vi "Launch Game.vi"() -> ()   [LabVIEW 2020]
uses:
  Main Reversi.vi
  Reversi.lvclass
panel:
  in  "Wait per Turn (ms)":u32=200 max=1000
  in  "Close":bool
  in  "Start":bool
  in  "Game Mode":T1(ring)=enum."Challenge Matches (All Players)"
  in  "Games Per Match":u32=1 min=1 max=1000
  # "Wait is changeable during the game."
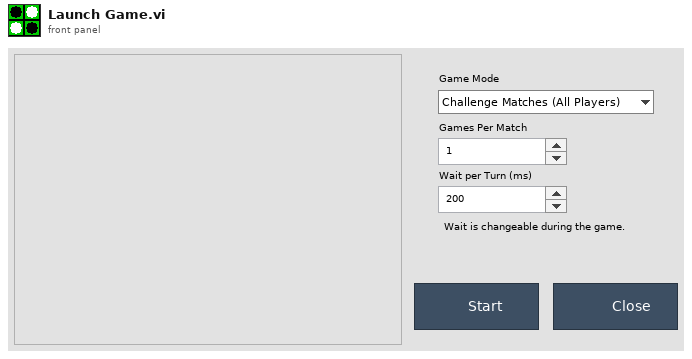
[diagram p1: front panel]
types:
  T1 = enum16{"One Game-Choose Players", "Challenge Matches (All Players)"}
  T2 = enum32{"Invalid", "Standard", "Closed", "Hidden", "Minimized", "Maximized"}
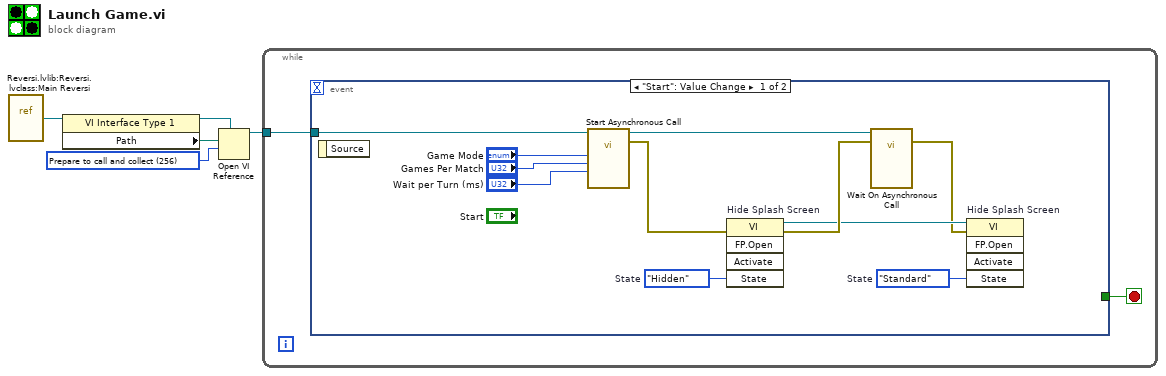
[diagram p0: block diagram]
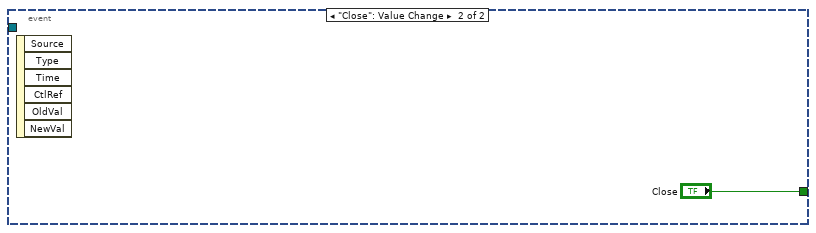
[diagram p2: hidden frame]
diagram:
  w1 = 256 items=["Record modifications"=1, "Open templates for editing"=2, "Prompt user to save"=4, "Prepare for reentrant run"=8, "Prompt to find missing subVIs"=16, "Hide loading dialog box"=32, "Enable simultaneous calls"=64, "Prepare to call and forget"=128, "Simultaneous call and forget"=192, "Prepare to call and collect"=256, "Simultaneous call and collect"=320]
  n1 = vi-ref "Reversi.lvlib:Reversi.lvclass:Main Reversi.vi"() -> (w5:refnum<vi>)
  n2 = property class="VI Interface Type 1"(reference=w5) -> (reference out=w3:refnum<vi>, "Path"=w4:path)  [unwired: 1 in, 1 out]
  n3 = Open VI Reference(type specifier VI Refnum (for type only)=w3, vi path=w4, options=w1) -> (vi reference=w2:refnum<vi>)  [unwired: 3 in, 1 out]
  n4 = while {
    tunnel: w2 -> [w7]
    stop <- w6 stop-if-true
    n5 = event shown="[0] \"Start\": Value Change" {
      selector: _ -> [_ _]
      dyn-events: _ -> [_ _]
      timeout: _ -> [_ _]
      tunnel: w7 -> [w18 _]
      tunnel: [_ "Close"] -> w6
      event "Start": Value Change {
        w10 = T2."Standard"  # State
        w13 = T2."Hidden"  # State
        n6 = event-data() -> ()  [unwired: 1 in, 1 out]
        n7 = call-by-ref "Start Asynchronous Call"(reference=w18, "Wait per Turn (ms)"="Wait per Turn (ms)", "Games Per Match"="Games Per Match", "Game Mode"="Game Mode") -> (reference out=w12:refnum<vi>, error out=w14:errorcluster)  [unwired: 9 in, 1 out]
        n8 = invoke on="Hide Splash Screen" class="VI" method="FP.Open"(error in=w14, "State"=w13) -> (reference out=w9:refnum<vi>, error out=w11:errorcluster)  [unwired: 3 in, 3 out]
        n9 = call-by-ref "Wait On Asynchronous Call"(reference=w12, error in=w11) -> (error out=w8:errorcluster)  [unwired: 11 in, 2 out]
        n10 = invoke on="Hide Splash Screen" class="VI" method="FP.Open"(reference=w9, error in=w8, "State"=w10) -> ()  [unwired: 2 in, 5 out]
      }
      event "Close": Value Change {
        n11 = event-data() -> ()  [unwired: 1 in, 6 out]
      }
    }
  }
